vi "Not16.vi"(3 "in":bool[](array[boolean])=[FALSE, FALSE, FALSE, FALSE, FALSE, FALSE, FALSE, FALSE, FALSE, FALSE, FALSE, FALSE, FALSE, FALSE, FALSE, FALSE]) -> (1 "out":bool[](array[boolean]))   [LabVIEW 2014]
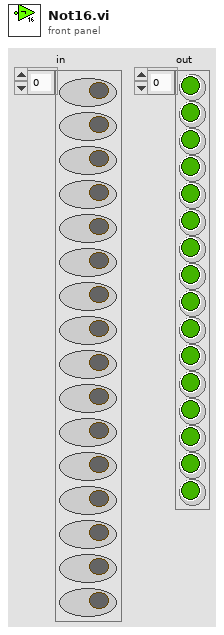
[diagram p1: front panel]
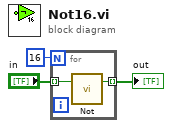
[diagram p0: block diagram]
diagram:
  n1 = for {
    N: 16 -> [_]
    tunnel: "in" -> [w5] mode=indexing
    tunnel: [w4] -> w2 mode=indexing
    n2 = call "Not.vi"("in"=w5) -> ("out"=w4:bool)  [unwired: 2 in]
  }
  "out" <- w2
